vi "PicoScope5000aExampleBlock.vi"() -> ()   [LabVIEW 2013]
panel:
  in  "Serial Number":string
  in  "Open using Serial Number":bool
  out "Channel B":i16[](graph)
  in  "Channel B Settings":T1={"Enabled"=FALSE, "Coupling"=1, "Range"=6, "Analogue Offset"=0.0} {"Range" items=["10 mV", "20 mV", "50 mV", "100 mV", "200 mV", "500 mV", "1 V", "2 V", "5 V", "10 V", "20 V", "50 V ", "100 V"]; "Coupling" items=["AC", "DC"]}
  in  "Resolution":i32(ring) items=["8-bit", "12-bit", "14-bit", "15-bit (max. 2 ch.)", "16-bit (max. 1 ch.)"]
  in  "PS5X4XA/B devices \nUSB Powered":bool=TRUE
  in  "Trigger Settings":T2={"Trigger Enabled"=TRUE, "Trigger Source"=enum."Channel A", "Trigger Threshold (16-bit counts)"=16384, "Trigger Direction"=2, "Trigger Delay (samples)"=0, "Auto Trigger Time (ms)"=0} {"Trigger Direction" items=["Rising"=2, "Falling"=3]}
  in  "Acquisition Settings":T3={"preTriggerSamples"=512, "postTriggerSamples"=512, "timebase"=127, "Down-Sample Mode"=0, "Down Sample Ratio"=1, "Four Channel Device"=FALSE} {"Down Sample Ratio" min=1 step=1; "Down-Sample Mode" items=["None"=0, "Aggregate"=1, "Decimate"=2, "Average"=4]}
  in  "Channel A Settings":T1={"Enabled"=TRUE, "Coupling"=1, "Range"=6, "Analogue Offset"=0.0} {"Range" items=["10 mV", "20 mV", "50 mV", "100 mV", "200 mV", "500 mV", "1 V", "2 V", "5 V", "10 V", "20 V", "50 V ", "100 V"]; "Coupling" items=["AC", "DC"]}
  in  "stop":bool
  out "Channel A":i16[](graph)
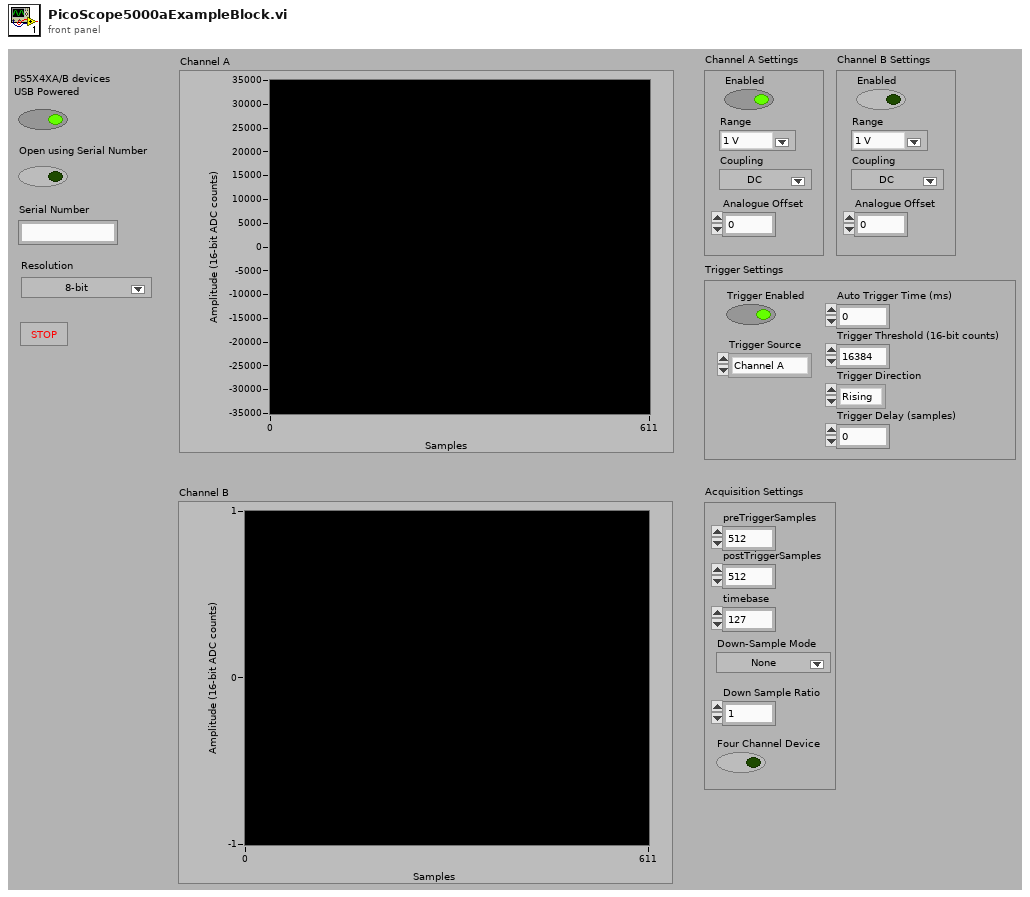
[diagram p1: front panel]
types:
  T1 = cluster{"Enabled":bool, "Coupling":i16, "Range":u16, "Analogue Offset":sgl}
  T2 = cluster{"Trigger Enabled":bool, "Trigger Source":enum16{"Channel A", "Channel B", "Channel C", "Channel D", "Ext."}, "Trigger Threshold (16-bit counts)":i16, "Trigger Direction":u16, "Trigger Delay (samples)":u32, "Auto Trigger Time (ms)":i16}
  T3 = cluster{"preTriggerSamples":u32, "postTriggerSamples":u32, "timebase":u32, "Down-Sample Mode":i32, "Down Sample Ratio":u32, "Four Channel Device":bool}
  T4 = cluster{"Channel D Buffer":i16[], "Channel C Buffer":i16[], "Channel B Buffer":i16[], "Channel A Buffer":i16[]}
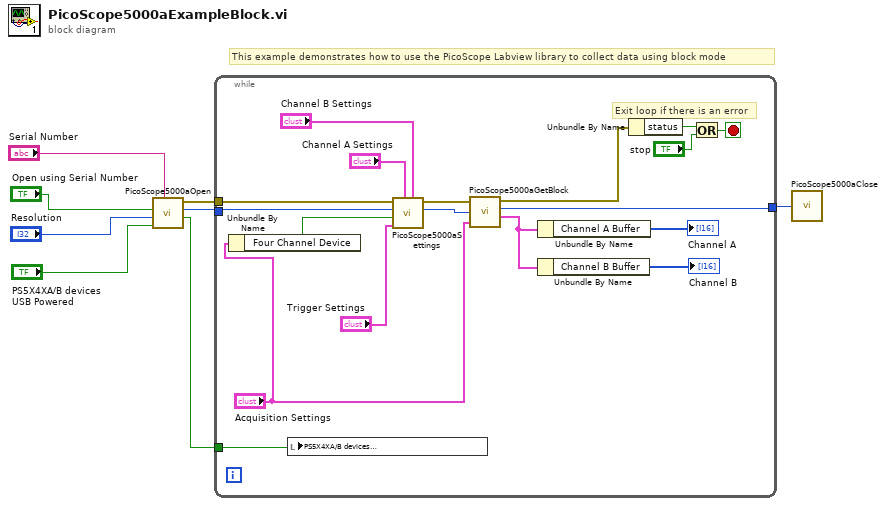
[diagram p0: block diagram]
diagram:
  # "This example demonstrates how to use the PicoScope Labview library to collect data using block mode"
  n1 = call "PicoScope5000aOpen.vi"("Serial Number"="Serial Number", "USB Powered Selection"="PS5X4XA/B devices \nUSB Powered", "Resolution"="Resolution", "Use Serial Number"="Open using Serial Number") -> ("USB Powered Indication"=w5:bool, "handle"=w6:i16, "error out"=w7:errorcluster)  [unwired: 2 in, 1 out]
  n2 = while {
    tunnel: w6 -> [w23]
    tunnel: w7 -> [w22]
    tunnel: [w21] -> w8
    tunnel: w5 -> [w14]
    stop <- w26 stop-if-true
    # "Exit loop if there is an error"
    n3 = Unbundle By Name("Acquisition Settings") -> ("Four Channel Device"=w9:bool)
    n4 = local write "PS5X4XA/B devices \nUSB Powered"(w14) -> ()
    n5 = call "PicoScope5000aSettings.vi"("Channel B Settings"="Channel B Settings", "Channel A Settings"="Channel A Settings", "Trigger Settings"="Trigger Settings", "Four Channel Device?"=w9, "handle in"=w23, "error in"=w22) -> ("handle out"=w19:i16, "error out"=w18:errorcluster)  [unwired: 4 in]
    n6 = call "PicoScope5000aGetBlock.vi"("error in"=w18, "handle in"=w19, "Acquisition Settings"="Acquisition Settings") -> ("error out"=w20:errorcluster, "handle out"=w21:i16, "Buffers (Max or non-aggregated)"=w12:T4)  [unwired: 3 in, 2 out]
    n7 = Unbundle By Name(w12) -> ("Channel A Buffer"=→"Channel A":i16[])
    n8 = Unbundle By Name(w12) -> ("Channel B Buffer"=→"Channel B":i16[])
    n9 = Unbundle By Name(w20) -> ("status"=w17:bool)
    n10 = Or(x=w17, y="stop") -> (x .or. y?=w26:bool)
  }
  n11 = call "PicoScope5000aClose.vi"("handle"=w8) -> ()
